vi "Set Adapter.vi"(8 "error in (no error)":errorcluster, 10 "Specific Execution Adapter":refnum<class "I Execution Adapter.lvclass">, 11 "Execution Service in":refnum<class "Execution Service.lvclass">) -> (0 "error out":errorcluster, 3 "Execution Service out":refnum<class "Execution Service.lvclass">)   [LabVIEW 2026, in "Execution Service.lvclass"]
uses:
  Execution Service.lvclass
  Interfaces/I Execution Adapter/I Execution Adapter.lvclass
  Execution Service.lvclass/Execution Service.ctl
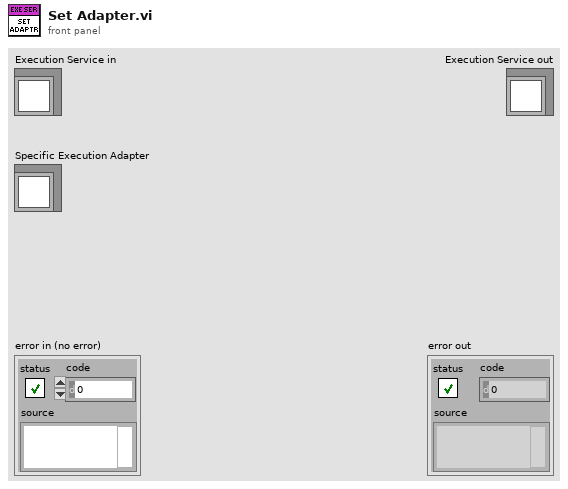
[diagram p1: front panel]
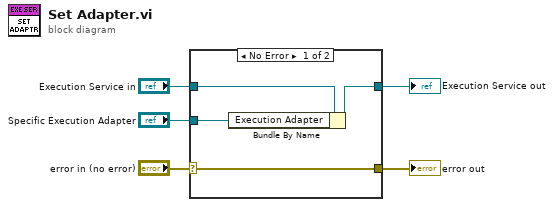
[diagram p0: block diagram]
diagram:
  n1 = case shown="No Error" "error in (no error)" {
    selector: "error in (no error)" -> [w6 w10]
    tunnel: "Execution Service in" -> [w9 w11]
    tunnel: "Specific Execution Adapter" -> [w8 _]
    tunnel: [w7 w11] -> w3
    tunnel: [w6 w10] -> w1
    frame No Error {
      n2 = Bundle By Name(cluster=w9, "Execution Adapter"=w8) -> (w7:refnum<class "Execution Service.lvclass">)
    }
    frame Error {
    }
  }
  "Execution Service out" <- w3
  "error out" <- w1
